vi "NIDCPower_channel_ganging - output connected.vi"(8 "error in (no error)":errorcluster, 9 "output enabled":bool=TRUE caption="output connected", 11 "Ganged Session In":T1) -> (0 "error out":errorcluster, 3 "Ganged Session Out":T1)   [LabVIEW 2021]
uses:
  ctl/NIDCPower_channel_ganging - ctl - ganged session.ctl
  ctl/NIDCPower_channel_ganging - ctl - ganged config.ctl
  ctl/NIDCPower_channel_ganging - ctl - channel mode.ctl
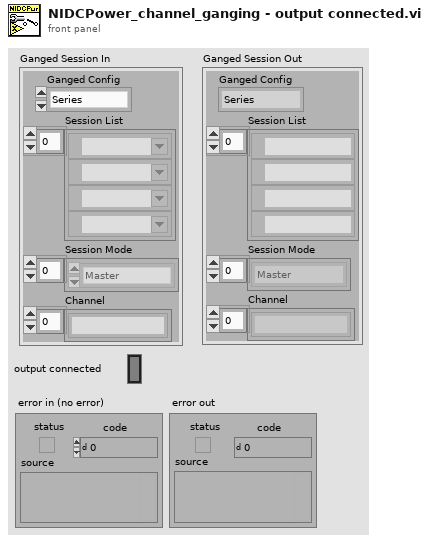
[diagram p1: front panel]
types:
  T1 = typedef "NIDCPower_channel_ganging - ctl - ganged session.ctl" = cluster{"Ganged Config":T2, "Session List":refnum<k15>[], "Session Mode":T3[], "Channel":string[]}
  T2 = typedef "NIDCPower_channel_ganging - ctl - ganged config.ctl" = enum32{"Series", "Parallel", "Manual"}
  T3 = typedef "NIDCPower_channel_ganging - ctl - channel mode.ctl" = enum32{"Master", "Slave", "Slave - Inverted"}
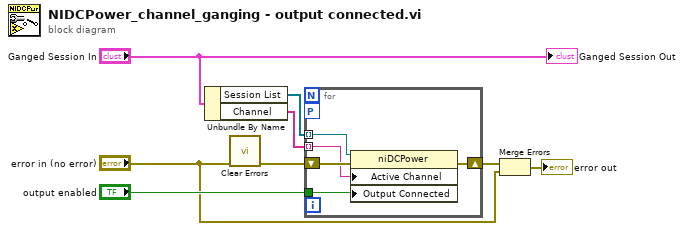
[diagram p0: block diagram]
diagram:
  n1 = Unbundle By Name("Ganged Session In") -> ("Session List"=w6:refnum<k15>[], "Channel"=w5:string[])
  n2 = call <vilib>:"Clear Errors.vi"("error in (no error)"="error in (no error)") -> ("error out"=w4:errorcluster)  [unwired: 5 in, 1 out]
  n3 = for {
    shift-right: [w10] -> w2
    shift-left: w4 -> [w12]
    tunnel: w6 -> [w13] mode=indexing
    tunnel: "output enabled" -> [w11]
    workers-P: _ -> [_]
    tunnel: w5 -> [w9] mode=indexing
    n4 = property class="niDCPower"(reference=w13, error in=w12, "Active Channel"=w9, "Output Connected"=w11) -> (error out=w10:errorcluster)  [unwired: 1 out]
  }
  n5 = Merge Errors(w2, "error in (no error)") -> (→"error out":errorcluster)
  "Ganged Session Out" <- "Ganged Session In"
